vi "Main.vi"() -> ()   [LabVIEW 2021]
uses:
  TypeDef/StateMachine.ctl
  TypeDef/SelectInstrument.ctl
  <vilib>/Utility/file.llb/Write Delimited Spreadsheet (string).vi
panel:
  out "Calculating":bool
  out "Points on graph":cluster{dbl[], dbl[]}
  in  "Choose path to save file (.csv)":path
  in  "Save to Excel":bool
  out "Commutator":refnum<visa-resource-name>
  out "Multimeter":refnum<visa-resource-name>
  out "Power Source":refnum<visa-resource-name>
  in  "Number of meas. points":i32=10 min=10 max=30 step=1
  out "I c. [A]":dbl
  out "U c. [V]":dbl
  out "XY Graph":cluster{"Voltage Array":dbl[], "Ic Array":dbl[]}(graph)
  in  "Stop":bool
  in  "Measurments":i32(listbox)
  out "Measurments":i32
  in  "Max. transistor power":dbl=5.0 caption="P [mW]" min=5.0 max=150.0 step=1.0
  in  "Restart":bool
  in  "Measure":bool
  in  "PSU A or B":bool
  in  "Voltage B":dbl(knob) caption="U [V]" min=0.0 max=25.0 step=0.01 scale=0.0..25.0 scale format="%#.3f"
  out "HP34401":dbl format="%#_5f"
  in  "Current  A":dbl(knob) caption="I [mA]" min=0.0 max=50.0 step=0.01 scale=0.0..50.0 scale format="%#.3f"
  # "Octocoupler CNY17"
  # "Max 10"
  # "A"
  # "B"
  # "X"
  # "Ch. 6"
  # "Ch. 7"
  # "Y"
  # "Scheme"
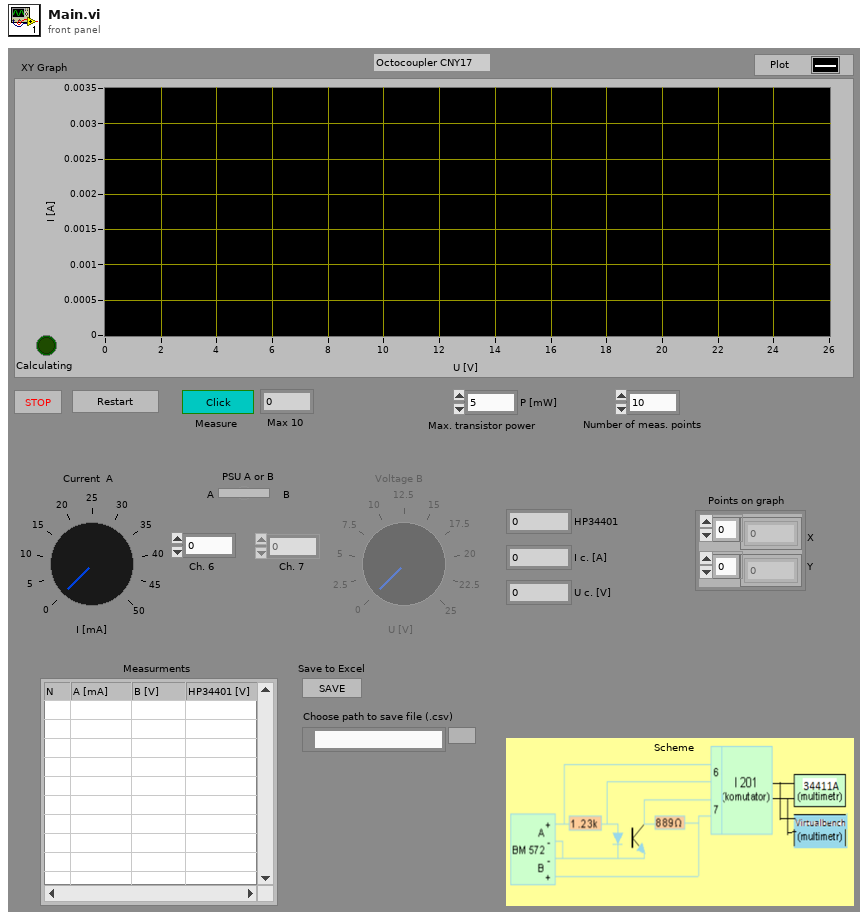
[diagram p1: front panel]
types:
  T1 = typedef "StateMachine.ctl" = enum16{"INIT", "Restart", "Idle", "Measure", "Create Listbox", "Draw Graph", "Save", "Stop"}
  T2 = enum8{"Enabled", "Disabled", "Disabled and Grayed Out"}
  T3 = typedef "SelectInstrument.ctl" = string
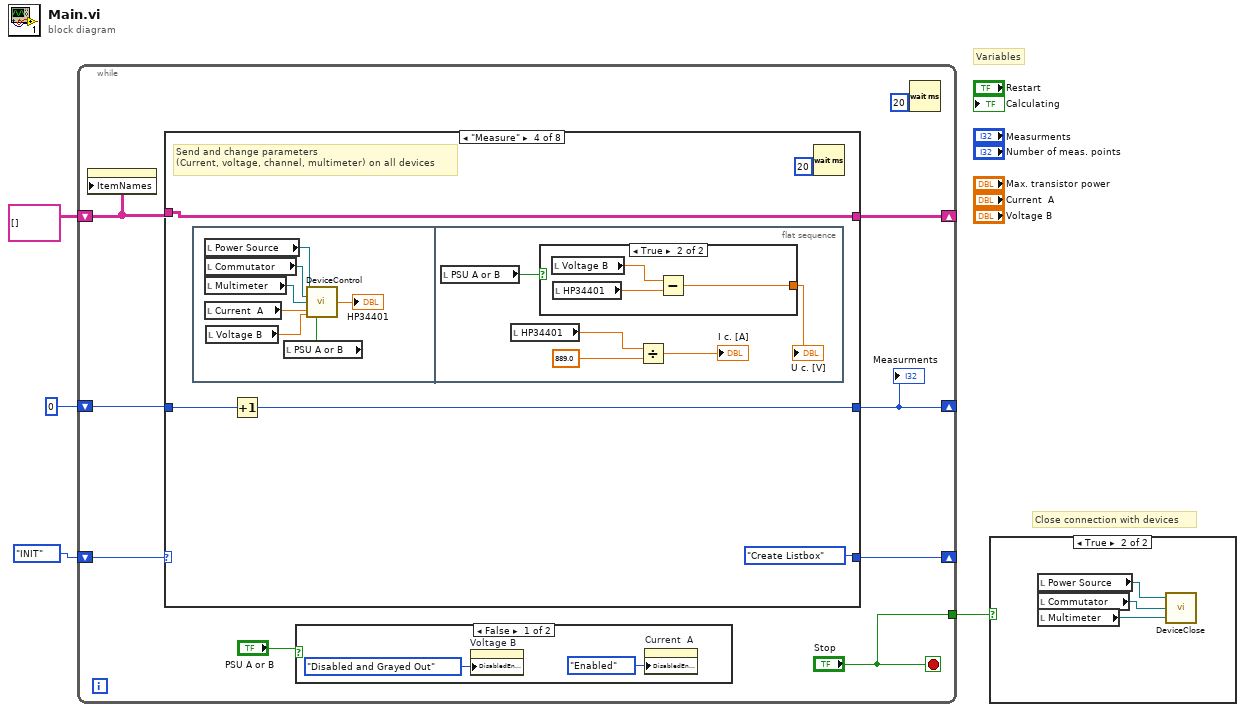
[diagram p0: block diagram]
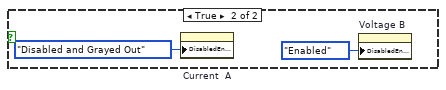
[diagram p3: hidden frame]
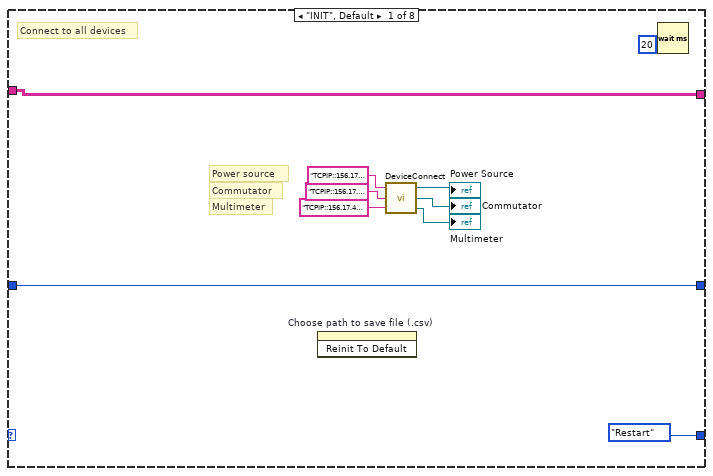
[diagram p4: hidden frame]
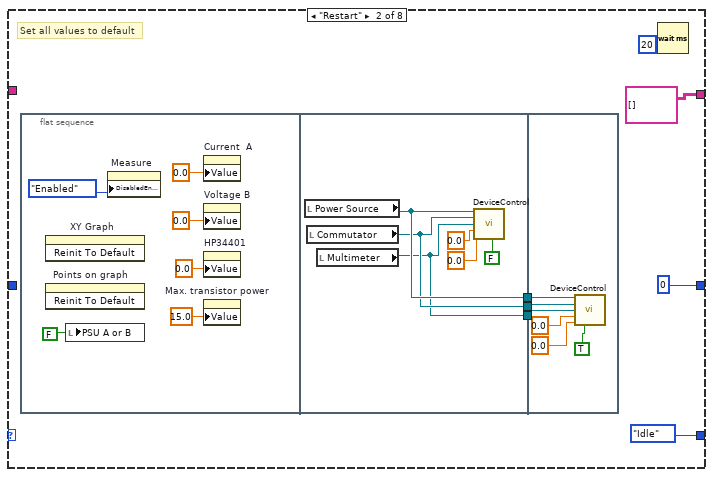
[diagram p5: hidden frame]
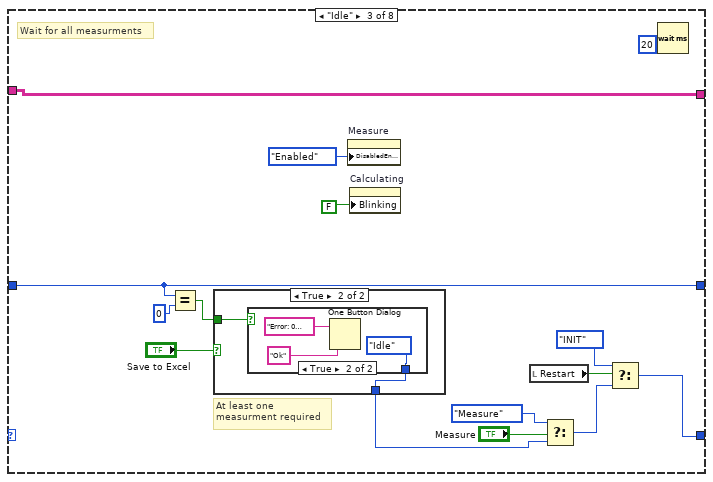
[diagram p6: hidden frame]
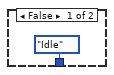
[diagram p7: hidden frame]
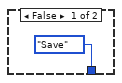
[diagram p8: hidden frame]
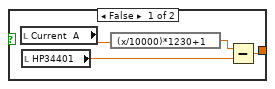
[diagram p9: hidden frame]
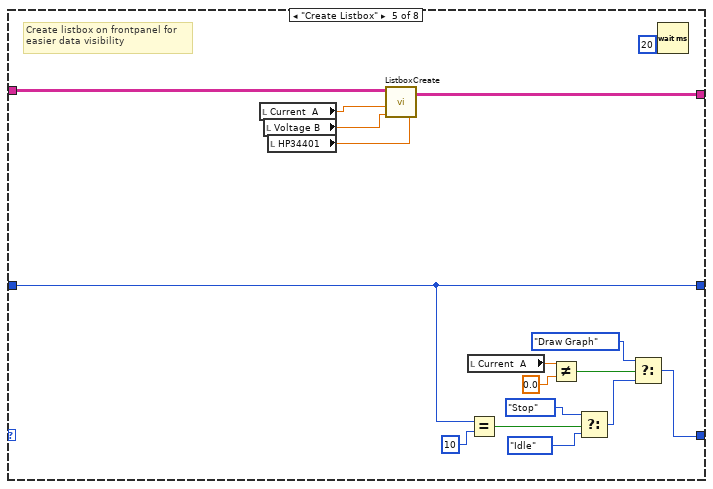
[diagram p10: hidden frame]
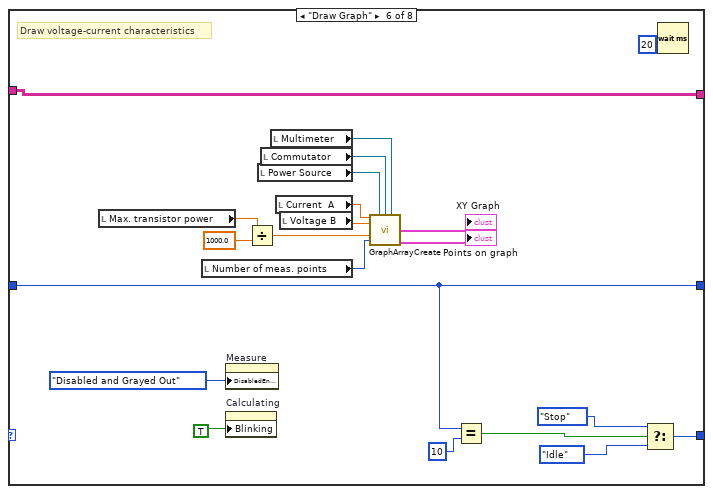
[diagram p11: hidden frame]
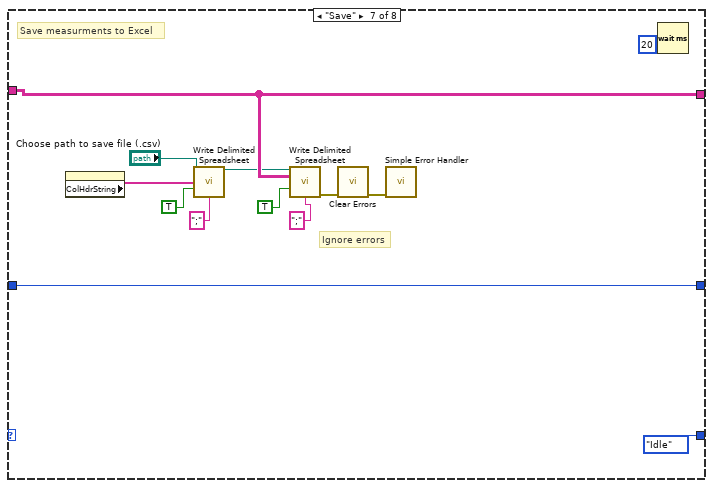
[diagram p12: hidden frame]
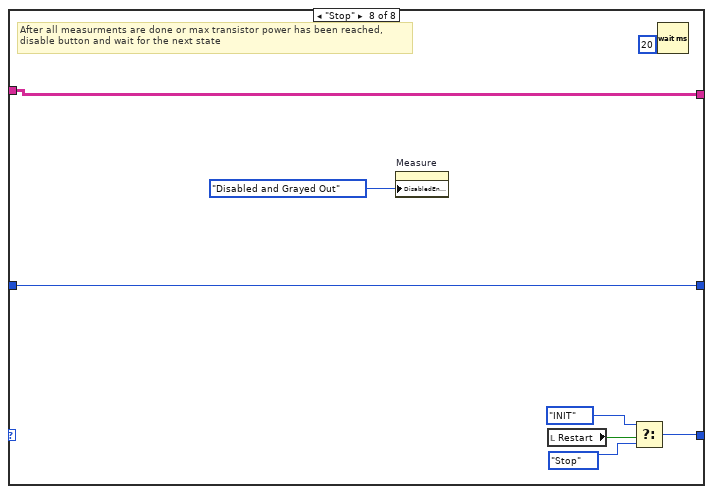
[diagram p13: hidden frame]
diagram:
  # "Variables"
  # "Close connection with devices"
  n1 = while {
    shift-right: [w13] -> _
    shift-left: StateMachine."INIT" -> [w6]
    shift-right: [w10] -> _
    shift-left: 0 -> [w11]
    shift-right: [w9] -> _
    shift-left: string[][] [] -> [w8]
    tunnel: ["Stop"] -> w1
    stop <- "Stop" stop-if-true
    n2 = property on="Measurments" class="MCListbox (strict)"("ItemNames"=w8) -> ()  [unwired: 2 in, 2 out]
    n3 = case shown="\"Measure\"" w6 {
      tunnel: [StateMachine."Restart" StateMachine."Idle" w62 StateMachine."Create Listbox" w108 w134 StateMachine."Idle" w152] -> w13
      tunnel: w11 -> [w25 _ w59 w77 w102 w131 w149 w156]
      tunnel: [w25 0 w59 w78 w102 w131 w149 w156] -> w10
      tunnel: w8 -> [w26 _ w60 w75 w113 w133 w147 w150]
      tunnel: [w26 string[][] [] w60 w75 w112 w133 w147 w150] -> w9
      frame "INIT", Default {
        # "Connect to all devices"
        # "Multimeter"
        # "Commutator"
        # "Power source"
        n4 = invoke on="Choose path to save file (.csv)" class="Path" method="Reinit To Default"() -> ()  [unwired: 3 in, 3 out]
        n5 = call "DeviceConnect.vi"("VISA resource name 3"=T3 "TCPIP::156.17.45.35::inst20::INSTR" ("Select_Instrument"), "VISA resource name 2"=T3 "TCPIP::156.17.45.35::inst19::INSTR" ("Select_Instrument"), "VISA resource name"=T3 "TCPIP::156.17.45.35::inst17::INSTR" ("Select_Instrument")) -> ("Multimeter"=→"Multimeter":refnum<visa-resource-name>, "Commutator"=→"Commutator":refnum<visa-resource-name>, "Power Source"=→"Power Source":refnum<visa-resource-name>)
        n6 = Wait (ms)(milliseconds to wait=u32 20) -> ()  [unwired: 1 out]
      }
      frame "Restart" {
        # "Set all values to default"
        n7 = flat-sequence {
          tunnel: [w43] -> w30
          tunnel: [w42] -> w29
          tunnel: [w41] -> w28
          tunnel: w30 -> [w49]
          tunnel: w29 -> [w48]
          tunnel: w28 -> [w47]
          frame #0 {
            n8 = invoke on="XY Graph" class="XYGraph (strict)" method="Reinit To Default"() -> ()  [unwired: 3 in, 3 out]
            n9 = invoke on="Points on graph" class="Clust (strict)" method="Reinit To Default"() -> ()  [unwired: 3 in, 3 out]
            n10 = local write "PSU A or B"(FALSE ("PSU A or B")) -> ()
            n11 = property on="Measure" class="Bool (strict)"("DisabledEnum"=T2."Enabled" ("Disabled")) -> ()  [unwired: 2 in, 2 out]
            n12 = property on="Current  A" class="Knob (strict)"("Value"=0.0 ("Current  A")) -> ()  [unwired: 2 in, 2 out]
            n13 = property on="Voltage B" class="Knob (strict)"("Value"=0.0 ("Current B")) -> ()  [unwired: 2 in, 2 out]
            n14 = property on="HP34401" class="DigNum (strict)"("Value"=0.0 ("Current B")) -> ()  [unwired: 2 in, 2 out]
            n15 = property on="Max. transistor power" class="DigNum (strict)"("Value"=15.0 ("Max. transistor power")) -> ()  [unwired: 2 in, 2 out]
          }
          frame #1 {
            n16 = local read "Power Source"() -> (w43:refnum<visa-resource-name>)
            n17 = local read "Commutator"() -> (w42:refnum<visa-resource-name>)
            n18 = local read "Multimeter"() -> (w41:refnum<visa-resource-name>)
            n19 = call "DeviceControl.vi"("Power Source"=w43, "Commutator"=w42, "Multimeter"=w41, "Current A"=0.0, "Voltage  B"=0.0, "PSU A or B"=FALSE) -> ()  [unwired: 9 in, 1 out]
          }
          frame #2 {
            n20 = call "DeviceControl.vi"("Power Source"=w49, "Commutator"=w48, "Multimeter"=w47, "Current A"=0.0, "Voltage  B"=0.0, "PSU A or B"=TRUE) -> ()  [unwired: 9 in, 1 out]
          }
        }
        n21 = Wait (ms)(milliseconds to wait=u32 20) -> ()  [unwired: 1 out]
      }
      frame "Idle" {
        # "At least one\nmeasurment required"
        # "Wait for all measurments"
        n22 = Equal?(x=w59, y=0) -> (x = y?=w55:bool)
        n23 = case shown="True" "Save to Excel" {
          tunnel: [StateMachine."Idle" w69] -> w57
          tunnel: w55 -> [_ w70]
          frame False {
          }
          frame True {
            n24 = case shown="True" w70 {
              tunnel: [StateMachine."Save" StateMachine."Idle"] -> w69
              frame False {
              }
              frame True {
                n25 = One Button Dialog(message="Error: 0 measurments", button name ("OK")="Ok") -> ()  [unwired: 1 out]
              }
            }
          }
        }
        n26 = property on="Measure" class="Bool (strict)"("DisabledEnum"=T2."Enabled" ("Disabled")) -> ()  [unwired: 2 in, 2 out]
        n27 = property on="Calculating" class="Bool (strict)"("Blinking"=FALSE) -> ()  [unwired: 2 in, 2 out]
        n28 = local read "Restart"() -> (w64:bool)
        n29 = Select(t=StateMachine."Measure", s="Measure", f=w57) -> (s? t:f=w61:T1)
        n30 = Select(t=StateMachine."INIT", s=w64, f=w61) -> (s? t:f=w62:T1)
        n31 = Wait (ms)(milliseconds to wait=u32 20) -> ()  [unwired: 1 out]
      }
      frame "Measure" {
        # "Send and change parameters \n(Current, voltage, channel, multimeter) on all devices"
        n32 = flat-sequence {
          frame #0 {
            n33 = local read "Power Source"() -> (w81:refnum<visa-resource-name>)
            n34 = local read "Commutator"() -> (w82:refnum<visa-resource-name>)
            n35 = local read "Multimeter"() -> (w83:refnum<visa-resource-name>)
            n36 = local read "Current  A"() -> (w85:dbl)
            n37 = local read "Voltage B"() -> (w84:dbl)
            n38 = local read "PSU A or B"() -> (w86:bool)
            n39 = call "DeviceControl.vi"("Power Source"=w81, "Commutator"=w82, "Multimeter"=w83, "Current A"=w85, "Voltage  B"=w84, "PSU A or B"=w86) -> ("HP34401"=→"HP34401":dbl)  [unwired: 9 in]
          }
          frame #1 {
            n40 = local read "PSU A or B"() -> (w88:bool)
            n41 = local read "HP34401"() -> (w91:dbl)
            n42 = case shown="True" w88 {
              tunnel: [w94 w96] -> w87
              frame False {
                n43 = local read "Current  A"() -> (w93:dbl)
                n44 = local read "HP34401"() -> (w95:dbl)
                n45 = expression code="(x/10000)*1230+1"(w93) -> (w92:dbl)
                n46 = Subtract(x=w92, y=w95) -> (x-y=w94:dbl)
              }
              frame True {
                n47 = local read "Voltage B"() -> (w97:dbl)
                n48 = local read "HP34401"() -> (w98:dbl)
                n49 = Subtract(x=w97, y=w98) -> (x-y=w96:dbl)
              }
            }
            "U c. [V]" <- w87
            n50 = Divide(x=w91, y=889.0) -> (x/y=→"I c. [A]":dbl)
          }
        }
        n51 = Increment(x=w77) -> (x+1=w78:i32)
        n52 = Wait (ms)(milliseconds to wait=u32 20) -> ()  [unwired: 1 out]
      }
      frame "Create Listbox" {
        # "Create listbox on frontpanel for\neasier data visibility"
        n53 = local read "Current  A"() -> (w115:dbl)
        n54 = local read "Voltage B"() -> (w114:dbl)
        n55 = local read "HP34401"() -> (w110:dbl)
        n56 = call "ListboxCreate.vi"("HP34401 input"=w110, "Current B"=w114, "Current  A"=w115, "Array input"=w113) -> ("Array output"=w112:string[][])  [unwired: 1 in]
        n57 = local read "Current  A"() -> (w99:dbl)
        n58 = Equal?(x=w102, y=10) -> (x = y?=w103:bool)
        n59 = Not Equal?(x=w99, y=0.0) -> (x != y?=w101:bool)
        n60 = Select(t=StateMachine."Stop", s=w103, f=StateMachine."Idle") -> (s? t:f=w105:T1)
        n61 = Select(t=StateMachine."Draw Graph", s=w101, f=w105) -> (s? t:f=w108:T1)
        n62 = Wait (ms)(milliseconds to wait=u32 20) -> ()  [unwired: 1 out]
      }
      frame "Draw Graph" {
        # "Draw voltage-current characteristics"
        n63 = local read "Max. transistor power"() -> (w122:dbl)
        n64 = local read "Number of meas. points"() -> (w116:i32)
        n65 = property on="Measure" class="Bool (strict)"("DisabledEnum"=T2."Disabled and Grayed Out" ("Disabled")) -> ()  [unwired: 2 in, 2 out]
        n66 = property on="Calculating" class="Bool (strict)"("Blinking"=TRUE ("Value (Signaling)")) -> ()  [unwired: 2 in, 2 out]
        n67 = Divide(x=w122, y=1000.0) -> (x/y=w123:dbl)
        n68 = local read "Power Source"() -> (w130:refnum<visa-resource-name>)
        n69 = local read "Commutator"() -> (w128:refnum<visa-resource-name>)
        n70 = local read "Multimeter"() -> (w129:refnum<visa-resource-name>)
        n71 = local read "Current  A"() -> (w117:dbl)
        n72 = local read "Voltage B"() -> (w127:dbl)
        n73 = call "GraphArrayCreate.vi"("Current A"=w117, "Power Source"=w130, "Commutator"=w128, "Multimeter"=w129, "Voltage  B"=w127, "Max. transistor power"=w123, "Number of meas. points"=w116) -> ("XY Graph"=→"XY Graph":cluster{"Voltage Array":dbl[], "Ic Array":dbl[]}, "Cluster"=→"Points on graph":cluster{dbl[], dbl[]})  [unwired: 7 in]
        n74 = Equal?(x=w131, y=10) -> (x = y?=w125:bool)
        n75 = Select(t=StateMachine."Stop", s=w125, f=StateMachine."Idle") -> (s? t:f=w134:T1)
        n76 = Wait (ms)(milliseconds to wait=u32 20) -> ()  [unwired: 1 out]
      }
      frame "Save" {
        # "Ignore errors"
        # "Save measurments to Excel"
        n77 = property on="Measurments" class="MCListbox (strict)"() -> ("ColHdrString"=w144:string[])  [unwired: 2 in, 2 out]
        n78 = call-poly <vilib>:"Write Delimited Spreadsheet.vi"("file path (dialog if empty)"="Choose path to save file (.csv)", "1D data"=w144, "append to file? (new file:F)"=TRUE, "delimiter (\\t)"=";" ("delimiter (\\t)")) -> ("new file path (Not A Path if cancelled)"=w143:path)  [unwired: 10 in, 1 out]
        n79 = call-poly <vilib>:"Write Delimited Spreadsheet.vi"("file path (dialog if empty)"=w143, "2D data"=w147, "append to file? (new file:F)"=TRUE, "delimiter (\\t)"=";" ("delimiter (\\t)")) -> ("error out"=w139:errorcluster)  [unwired: 10 in, 1 out]
        n80 = call <vilib>:"Clear Errors.vi"("error in (no error)"=w139) -> ("error out"=w138:errorcluster)  [unwired: 5 in, 1 out]
        n81 = call <vilib>:"Simple Error Handler.vi"("error in (no error)"=w138) -> ()  [unwired: 4 in, 5 out]
        n82 = Wait (ms)(milliseconds to wait=u32 20) -> ()  [unwired: 1 out]
      }
      frame "Stop" {
        # "After all measurments are done or max transistor power has been reached,\ndisable button and wait for the next state"
        n83 = property on="Measure" class="Bool (strict)"("DisabledEnum"=T2."Disabled and Grayed Out" ("Disabled")) -> ()  [unwired: 2 in, 2 out]
        n84 = local read "Restart"() -> (w151:bool)
        n85 = Select(t=StateMachine."INIT", s=w151, f=StateMachine."Stop") -> (s? t:f=w152:T1)
        n86 = Wait (ms)(milliseconds to wait=u32 20) -> ()  [unwired: 1 out]
      }
    }
    "Measurments" <- w10
    n87 = case shown="False" "PSU A or B" {
      frame False {
        n88 = property on="Voltage B" class="Knob (strict)"("DisabledEnum"=T2."Disabled and Grayed Out" ("Disabled")) -> ()  [unwired: 2 in, 2 out]
        n89 = property on="Current  A" class="Knob (strict)"("DisabledEnum"=T2."Enabled" ("Disabled")) -> ()  [unwired: 2 in, 2 out]
      }
      frame True {
        n90 = property on="Current  A" class="Knob (strict)"("DisabledEnum"=T2."Disabled and Grayed Out" ("Disabled")) -> ()  [unwired: 2 in, 2 out]
        n91 = property on="Voltage B" class="Knob (strict)"("DisabledEnum"=T2."Enabled" ("Disabled")) -> ()  [unwired: 2 in, 2 out]
      }
    }
    n92 = Wait (ms)(milliseconds to wait=u32 20) -> ()  [unwired: 1 out]
  }
  n93 = case shown="True" w1 {
    frame False {
    }
    frame True {
      n94 = local read "Power Source"() -> (w158:refnum<visa-resource-name>)
      n95 = local read "Commutator"() -> (w160:refnum<visa-resource-name>)
      n96 = local read "Multimeter"() -> (w159:refnum<visa-resource-name>)
      n97 = call "DeviceClose.vi"("Multimeter"=w159, "Commutator"=w160, "Power Source"=w158) -> ()
    }
  }
